vi "Write Global Debug Level.vi"(8 "error in (no error)":errorcluster, 10 "Debug Level":T1, 11 "Registry in":refnum<class "Registry.lvclass">) -> (0 "error out":errorcluster, 3 "Registry out":refnum<class "Registry.lvclass">)   [LabVIEW 2020, in "LV Logging.lvlib" / "Registry.lvclass"]
uses:
  Registry.lvclass
  Registry.lvclass/Registry.ctl
  Type Defs/Debug Level.ctl
  LV Logging.lvlib
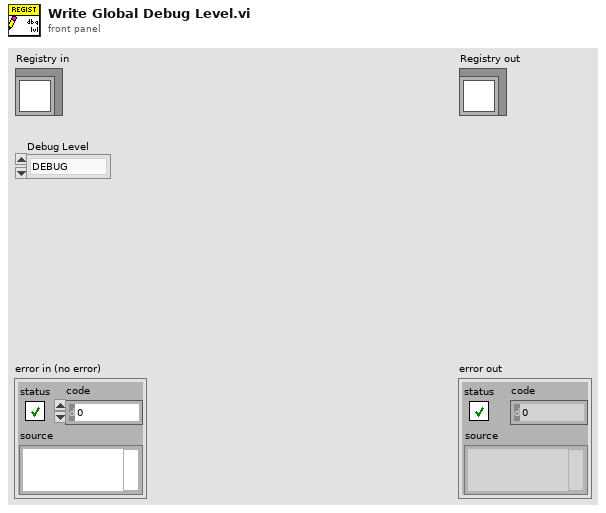
[diagram p1: front panel]
types:
  T1 = typedef "LV Logging.lvlib/Debug Level.ctl" = enum16{"DEBUG", "INFO", "WARN", "ERROR", "FATAL"}
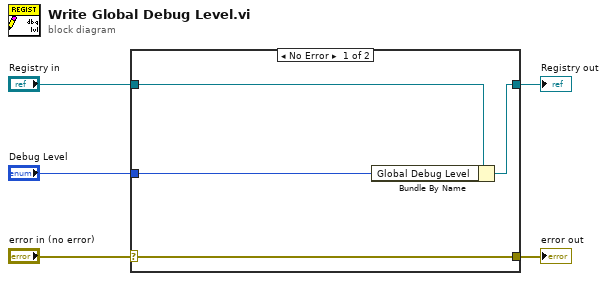
[diagram p0: block diagram]
diagram:
  n1 = case shown="No Error" "error in (no error)" {
    selector: "error in (no error)" -> [w9 w10]
    tunnel: [w9 w10] -> w4
    tunnel: [w7 w11] -> w2
    tunnel: "Registry in" -> [w8 w11]
    tunnel: "Debug Level" -> [w6 _]
    frame No Error {
      n2 = Bundle By Name(cluster=w8, "Global Debug Level"=w6) -> (w7:refnum<class "Registry.lvclass">)
    }
    frame Error {
    }
  }
  "error out" <- w4
  "Registry out" <- w2
